vi "Create Test Configuration.vi"() -> (0 "error out":errorcluster, 1 "Names":string[](array[string]), 2 "Line Array":T1[](array[typedef]), 3 "module":refnum<class "tag bus configurable plugin module configuration.lvclass">, 4 "Channels":refnum<class "TBM channel.lvclass">[](array[class]), 5 "instance identifier":string)   [LabVIEW 2013, in "Table Manager tests.lvlib"]
doc: "This VI creates the test configuration used in testing. BY default just creates one line with every datatype"
uses:
  Table Manager tests.lvlib
  module/configuration/tag bus configurable plugin module configuration.lvclass
  module/configuration/Line.ctl
  <vilib>/NI/Tag Bus Module Framework/channel/TBM channel.lvclass
  <vilib>/NI/Tag Bus Module Framework/channel/channel classification.ctl
  <vilib>/NI/Tag Bus/tag/default value polymorphs/write default value Single.vi
  <vilib>/NI/Configuration Framework/serializable configuration/NISE_CEF_serializable configuration.lvclass
  <vilib>/NI/Tag Bus/tag/tag descriptor.lvclass
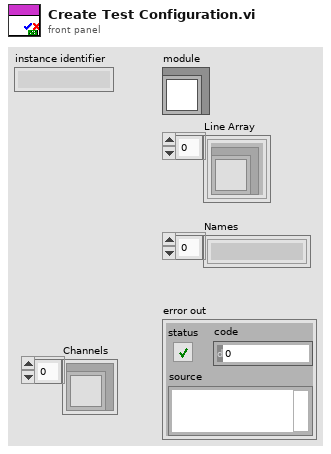
[diagram p1: front panel]
types:
  T1 = typedef "tag bus configurable plugin module configuration.lvclass/Line.ctl" = cluster{"channel":refnum<class "TBM channel.lvclass">}
  T2 = typedef "TBM channel.lvclass/channel classification.ctl" = enum16{"input data", "output data", "processing parameter", "processing result"}
  T3 = typedef "tag bus.lvlib/tag descriptor.lvclass/Data Type.ctl" = enum16{"Double", "Single", "I64", "I32", "I16", "I8", "U64", "U32", "U16", "U8", "Boolean", "String", "Array of Double", "Array of Single", "Array of I64", "Array of I32", "Array of I16", "Array of I8", "Array of U64", "Array of U32", "Array of U16", "Array of U8", "Array of Boolean", "Array of String"}
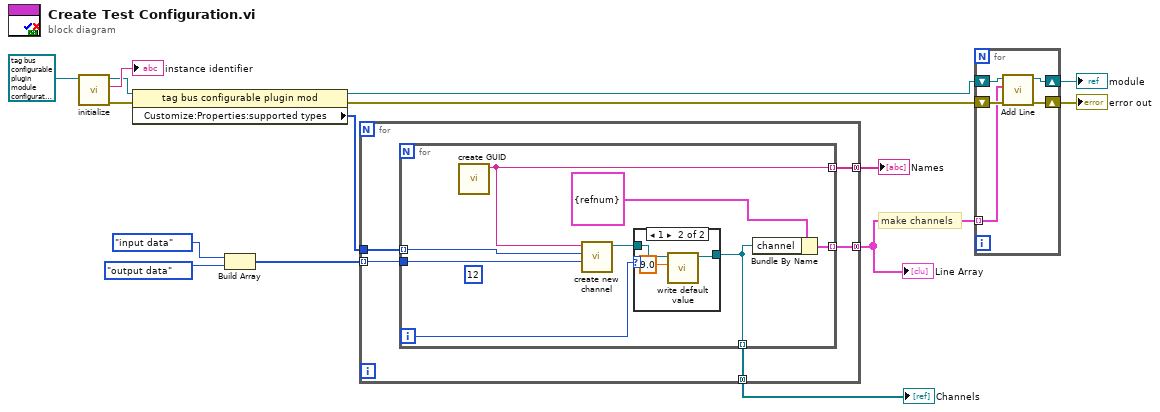
[diagram p0: block diagram]
diagram:
  # "make channels"
  n1 = call <vilib>:"initialize.vi"("configuration in"=refnum<class "tag bus configurable plugin module configuration.lvclass"> refnum ("tag bus configurable plugin module configuration")) -> ("error out"=w13:errorcluster, "identifier"=→"instance identifier":string, "configuration out"=w10:refnum<class "tag bus configurable plugin module configuration.lvclass">)  [unwired: 8 in]
  n2 = property class="tag bus configurable plugin mod"(reference=w10, error in=w13) -> (reference out=w5:refnum<class "tag bus configurable plugin module configuration.lvclass">, error out=w12:errorcluster, "Customize:Properties:supported types"=w6:T3[])
  n3 = Build Array(channel_classification."input data" ("channel classification"), channel_classification."output data" ("channel classification")) -> (w4:T2[])
  n4 = for {
    tunnel: w4 -> [w20] mode=indexing
    tunnel: [w18] -> w9 mode=concatenating
    tunnel: w6 -> [w19]
    tunnel: [w17] -> w11 mode=concatenating
    tunnel: [w16] -> w1 mode=concatenating
    n5 = for {
      tunnel: w20 -> [w28]
      tunnel: [w24] -> w18 mode=indexing
      tunnel: w19 -> [w27] mode=indexing
      tunnel: [w26] -> w17 mode=indexing
      tunnel: [w22] -> w16 mode=indexing
      i -> [w23]
      (unwired) 12
      n6 = call <vilib>:"create GUID.vi"() -> ("uuid"=w26:string)  [unwired: 10 in, 1 out]
      n7 = call <vilib>:"create new channel.vi"("channel classification"=w28, "data type"=w27, "channel name"=w26) -> ("channel"=w21:refnum<class "TBM channel.lvclass">)  [unwired: 8 in]
      n8 = case shown="1" w23 {
        tunnel: [w29 w31] -> w22
        tunnel: w21 -> [w29 w32]
        frame 0, Default {
        }
        frame 1 {
          n9 = call-poly <vilib>:"write default value.vi"("default value"=sgl 9.0, "system tag in"=w32) -> ("system tag out"=w31:refnum<class "TBM channel.lvclass">)  [unwired: 8 in, 1 out]
        }
      }
      n10 = Bundle By Name(cluster=T1 {"channel"=refnum} ("Line"), "channel"=w22) -> (w24:T1)
    }
  }
  "Names" <- w11
  "Line Array" <- w9
  "Channels" <- w1
  n11 = for {
    tunnel: w9 -> [w33] mode=indexing
    shift-right: [w36] -> w8
    shift-left: w5 -> [w37]
    shift-right: [w34] -> w15
    shift-left: w12 -> [w35]
    n12 = call "Add Line.vi"("error in"=w35, "Line"=w33, "tag bus configurable plugin module configuration in"=w37) -> ("error out"=w34:errorcluster, "tag bus configurable plugin module configuration out"=w36:refnum<class "tag bus configurable plugin module configuration.lvclass">)  [unwired: 7 in]
  }
  "error out" <- w15
  "module" <- w8
